vi "Get All LogicIOs.vi"(8 "error in (no error)":errorcluster, 11 "VacuumLine in":refnum<class "VacuumLine.lvclass">) -> (0 "error out":errorcluster, 1 "LogicIOs":refnum<class "LogicIO.lvclass">[](array[class]), 2 "labels":string[](array[string]), 3 "VacuumLine out":refnum<class "VacuumLine.lvclass">)   [LabVIEW 2016, in "Hardware.lvlib" / "VacuumLine.lvlib" / "VacuumLine.lvclass"]
uses:
  <userlib>/Common Components/Hardware/Abstract System/VacuumLine/VacuumLine/VacuumLine.lvclass
  <userlib>/Common Components/Hardware/LogicIO/LogicIO/LogicIO.lvclass
  <userlib>/Common Components/Hardware/Abstract System/VacuumLine/VacuumLine/VacuumLine.lvclass/VacuumLine.ctl
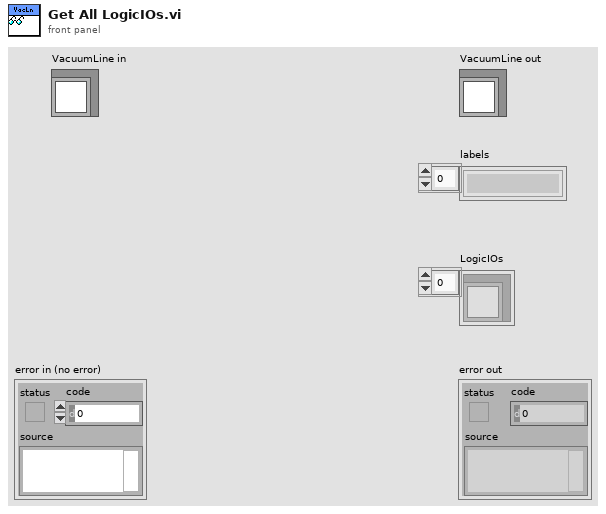
[diagram p1: front panel]
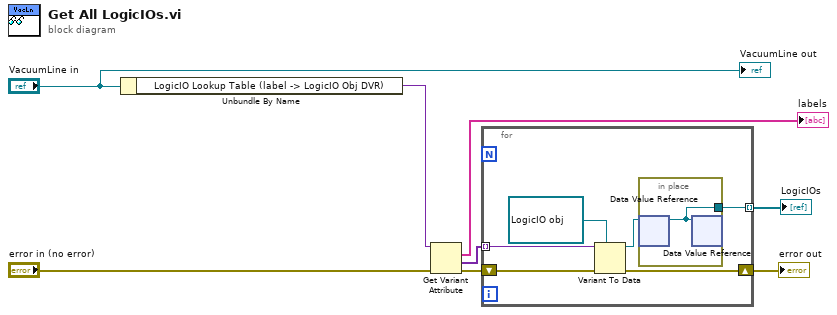
[diagram p0: block diagram]
diagram:
  n1 = Unbundle By Name("VacuumLine in") -> ("LogicIO Lookup Table (label -> LogicIO Obj DVR)"=w5:variant)
  n2 = Get Variant Attribute(Variant=w5, error in="error in (no error)") -> (names=→"labels":string[], values=w7:variant[], error out=w6:errorcluster)  [unwired: 2 in, 1 out]
  n3 = for {
    tunnel: w7 -> [w14] mode=indexing
    shift-right: [w12] -> w3
    shift-left: w6 -> [w13]
    tunnel: [w9] -> w2 mode=indexing
    n4 = Variant To Data(error in=w13, type=refnum<data-value> refnum ("data value reference"), Variant=w14) -> (data=w10:refnum<data-value>, error out=w12:errorcluster)
    n5 = in-place {
      in-place-border: [w15] -> w9
      n6 = in-place-dvr #1(w10) -> (w15:refnum<class "LogicIO.lvclass">)  [unwired: 1 out]
      n7 = in-place-dvr #1(w15) -> ()  [unwired: 2 out]
    }
  }
  "error out" <- w3
  "LogicIOs" <- w2
  "VacuumLine out" <- "VacuumLine in"
